vi "Read Data.vi"(8 "error in (no error)":errorcluster, 11 "Update Humidifier Output Data MSG in":refnum<class "Update Humidifier Output Data MSG.lvclass">) -> (0 "error out":errorcluster, 2 "Base Data Lib:Single_Array.lvclass":refnum<class "Single_Array.lvclass">, 3 "Update Humidifier Output Data MSG out":refnum<class "Update Humidifier Output Data MSG.lvclass">)   [LabVIEW 2014, in "Update Humidifier Output Data MSG.lvclass"]
uses:
  Update Humidifier Output Data MSG.lvclass
  reusable/Data/Array Data/Single 1-D/Single_Array.lvclass
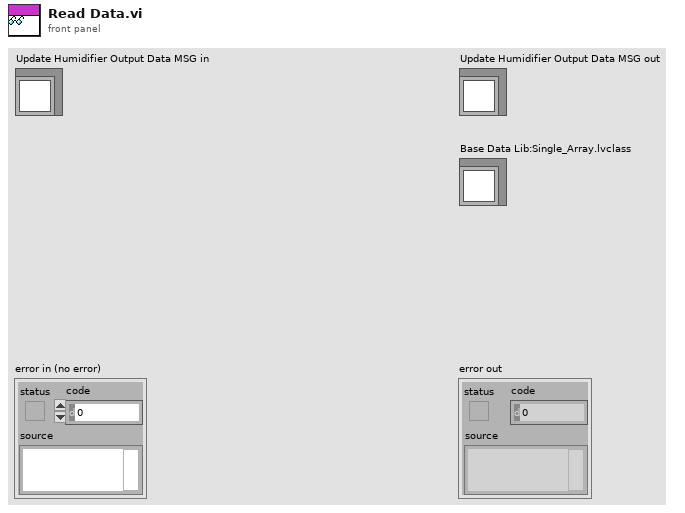
[diagram p1: front panel]
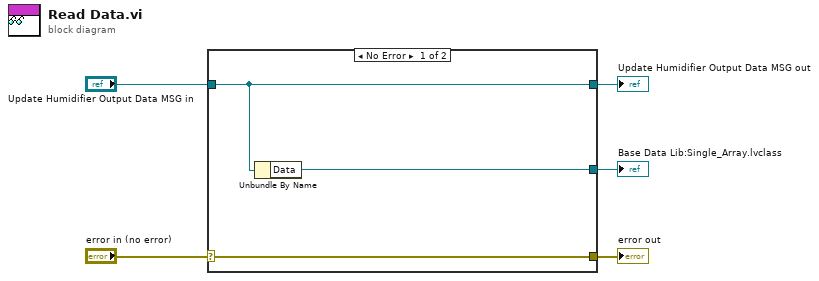
[diagram p0: block diagram]
diagram:
  n1 = case shown="No Error" "error in (no error)" {
    selector: "error in (no error)" -> [w8 w9]
    tunnel: [w8 w9] -> w4
    tunnel: [w7 w10] -> w2
    tunnel: "Update Humidifier Output Data MSG in" -> [w7 w10]
    tunnel: [w6 _] -> w1
    frame No Error {
      n2 = Unbundle By Name(w7) -> ("Data"=w6:refnum<class "Single_Array.lvclass">)
    }
    frame Error {
    }
  }
  "error out" <- w4
  "Update Humidifier Output Data MSG out" <- w2
  "Base Data Lib:Single_Array.lvclass" <- w1
